vi "CheckValueEqualsSetpoint.vi"(8 "Pressure tolerance %":dbl, 9 "PressureNewVal":dbl, 10 "Pressure":dbl) -> (0 "Current pressure status":string, 4 "PeqPSet ?":bool)   [LabVIEW 2019]
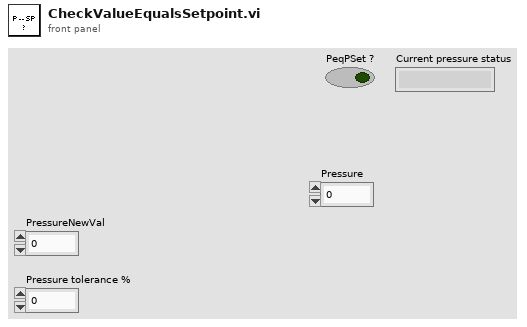
[diagram p1: front panel]
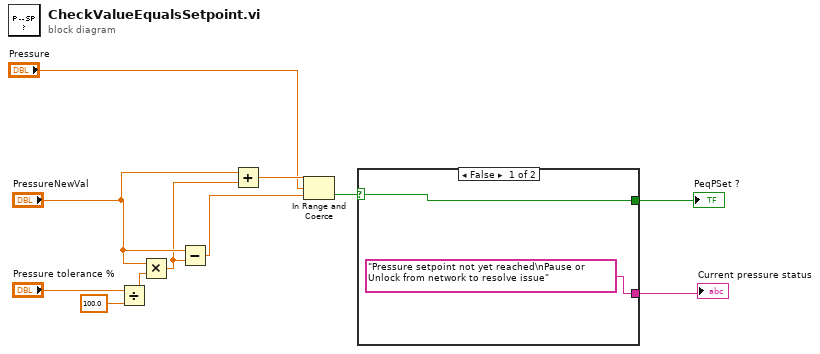
[diagram p0: block diagram]
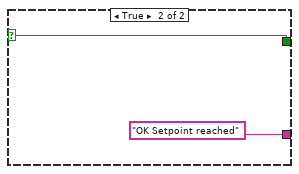
[diagram p2: hidden frame]
diagram:
  n1 = Divide(x="Pressure tolerance %", y=sgl 100.0) -> (x/y=w5:dbl)
  n2 = Multiply(x="PressureNewVal", y=w5) -> (x*y=w8:dbl)
  n3 = Subtract(x="PressureNewVal", y=w8) -> (x-y=w11:dbl)
  n4 = Add(x="PressureNewVal", y=w8) -> (x+y=w10:dbl)
  n5 = In Range and Coerce(upper limit=w10, x="Pressure", lower limit=w11) -> (In Range?=w4:bool)  [unwired: 1 out]
  n6 = case shown="False" w4 {
    selector: w4 -> [w13 w15]
    tunnel: [w13 w15] -> w3
    tunnel: ["Pressure setpoint not yet reached\nPause or Unlock from network to resolve issue" ("Current pressure status") "OK Setpoint reached" ("Current pressure status")] -> w2
    frame False {
    }
    frame True {
    }
  }
  "PeqPSet ?" <- w3
  "Current pressure status" <- w2
